vi "performance fg.vi"(1 "Input":T1, 2 "Menu":T2) -> (0 "Output":T1)   [LabVIEW 2013]
uses:
  typedefs/fg_typedef.ctl
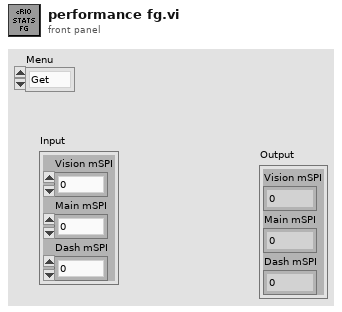
[diagram p1: front panel]
types:
  T1 = cluster{"Vision mSPI":u32, "Main mSPI":u32, "Dash mSPI":u32}
  T2 = typedef "fg_typedef.ctl" = enum16{"Get", "Set"}
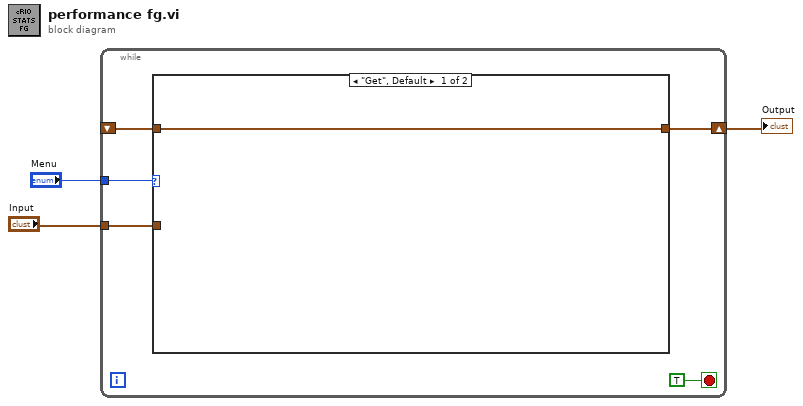
[diagram p0: block diagram]
diagram:
  n1 = while {
    tunnel: "Menu" -> [w7]
    shift-right: [w6] -> w2
    shift-left: _ -> [w5]
    tunnel: "Input" -> [w4]
    stop <- TRUE stop-if-true
    n2 = case shown="\"Get\", Default" w7 {
      tunnel: [w9 w10] -> w6
      tunnel: w5 -> [w9 _]
      tunnel: w4 -> [_ w10]
      frame "Get", Default {
      }
      frame "Set" {
      }
    }
  }
  "Output" <- w2
